vi "Decompose Build Trigger Cron String.vi"(11 "String":string) -> (3 "Cron Cluster":T1={"Day of Week"=enum."Everyday", "Hour"=1, "Enable?"=FALSE} {"Hour" min=0 max=23})   [LabVIEW 2014]
uses:
  Controls/Cron String - STYP.ctl
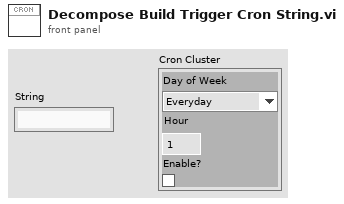
[diagram p1: front panel]
types:
  T1 = typedef "Cron String - STYP.ctl" = cluster{"Day of Week":enum16{"Everyday", "Sunday", "Monday", "Tuesday", "Wednesday", "Thursday", "Friday", "Saturday"}, "Hour":i32, "Enable?":bool}
  T2 = enum16{"Everyday", "Sunday", "Monday", "Tuesday", "Wednesday", "Thursday", "Friday", "Saturday"}
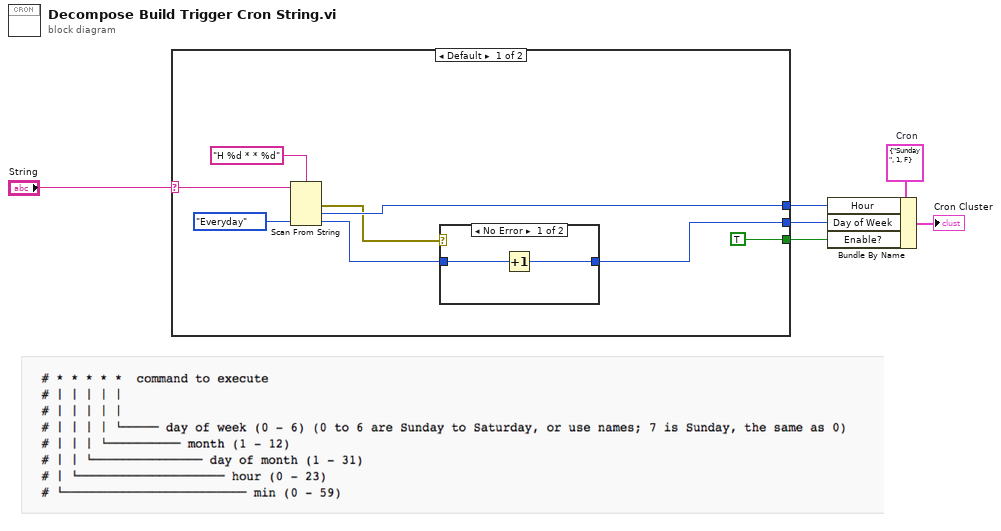
[diagram p0: block diagram]
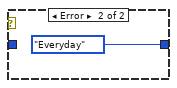
[diagram p2: hidden frame]
diagram:
  w5 = T1 {"Day of Week"=enum."Sunday", "Hour"=1, "Enable?"=FALSE}  # Cron
  n1 = case shown="Default" "String" {
    selector: "String" -> [w14 _]
    tunnel: [w9 _] -> w3
    tunnel: [w11 _] -> w4
    tunnel: [TRUE _] -> w1
    frame Default {
      n2 = Scan From String(format string="H %d * * %d", input string=w14, default 2=T2."Everyday" ("Day of Week")) -> (error out=w8:errorcluster, output 1=w11:i32, output 2=w7:T2)  [unwired: 3 in, 2 out]
      n3 = case shown="No Error" w8 {
        tunnel: [w15 T2."Everyday" ("Day of Week")] -> w9
        tunnel: w7 -> [w16 _]
        frame No Error {
          n4 = Increment(x=w16) -> (x+1=w15:T2)
        }
        frame Error {
        }
      }
    }
    frame "" {
    }
  }
  n5 = Bundle By Name(cluster=w5, "Hour"=w4, "Day of Week"=w3, "Enable?"=w1) -> (→"Cron Cluster":T1)
